vi "Test Cannot Open View Before Start.vi"(8 "error in (no error)":errorcluster, 11 "View Test In":refnum<class "View Dev Test.lvclass">) -> (0 "error out":errorcluster, 3 "View Test Out":refnum<class "View Dev Test.lvclass">)   [LabVIEW 2020, in "View Dev Test.lvclass"]
uses:
  View Dev Test.lvclass
  C:/Program Files (x86)/National Instruments/LabVIEW 2020/vi.lib/Astemes/LUnit/Test Case.lvclass
  source/Framework/Process/Process.lvclass/Process.ctl
  source/Framework/View/View.lvclass/View.ctl
  <vilib>/Astemes/LUnit/Test Case.lvclass/Test Case.ctl
  <vilib>/Astemes/LUnit/LUnit Assertion Result.lvclass/LUnit Assertion Result.ctl
  <vilib>/Astemes/LUnit/LUnit Test Case Result.lvclass/LUnit Test Case Result.ctl
  <vilib>/Astemes/LUnit/LUnit Method Result.lvclass/LUnit Method Result.ctl
  source/Framework/Process/Protected/Messaging/Enqueue Message.vi
  source/Framework/View/Public/Get View VI Reference.vi
  source/Framework/Process/Public/Lifecycle/Get Lifecycle State.vi
  <vilib>/Astemes/LUnit/Palette/Fail.vi
  <vilib>/Astemes/LUnit/Palette/Pass.vi
  <vilib>/Astemes/LUnit/Set Assertion Type.vi
  source/Framework/Process/Private/SubVIs/Handle Debug Data.vi
  source/Framework/Process/Protected/Messaging/Request Message.vi
  <vilib>/Utility/error.llb/Clear Errors.vi
  <vilib>/Astemes/LUnit/Add test result.vi
  <vilib>/Astemes/LUnit/LUnit Write Passed.vi
  <vilib>/Astemes/LUnit/LUnit Write Message.vi
  <vilib>/Astemes/LUnit/LUnit Write Description.vi
  <vilib>/Astemes/LUnit/LUnit Write Assertion Type.vi
  source/Framework/Logging/Log Debug.vi
  <vilib>/AdvancedString/1D String Array to Delimited String.vi
  <vilib>/Utility/High Resolution Relative Seconds.vi
  source/Framework/Process/Private/SubVIs/Enqueue Request Message.vi
  <vilib>/Astemes/LUnit/LUnit Record Assertion Result.vi
  <vilib>/Astemes/LUnit/LUnit Aggregate Assertion Results.vi
  <vilib>/Astemes/LUnit/Assertion Result/LUnit Read Status.vi
  <vilib>/Astemes/LUnit/LUnit Read Message.vi
  <vilib>/Astemes/LUnit/LUnit Read Description.vi
  <vilib>/Astemes/LUnit/Method Result/LUnit Merge Status.vi
  <vilib>/Astemes/LUnit/LUnit Concatenate result strings.vi
  source/Framework/View/View.lvclass
  C:/Git/astemes-triarc-framework/source/Framework/Process/Process.lvclass
  <vilib>/Utility/error.llb/Error Cluster From Error Code.vi
  source/Framework/Process/Public/Read Name.vi
  source/Framework/Process/Private/SubVIs/Wait for Response Message.vi
  <vilib>/Astemes/LUnit/LUnit Assertion Result.lvclass
  <vilib>/Astemes/LUnit/Test Case.lvclass
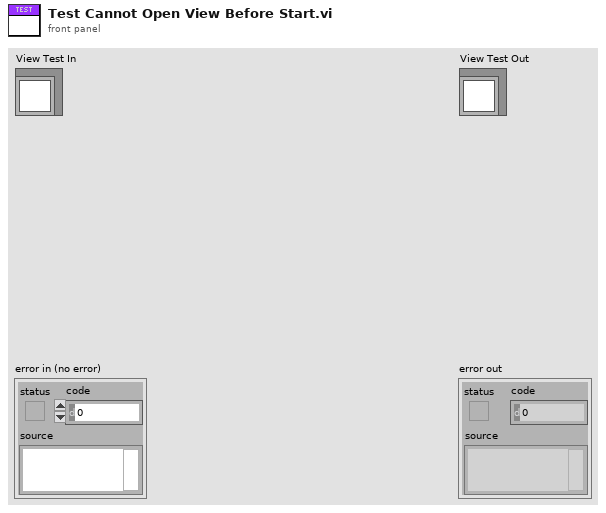
[diagram p1: front panel]
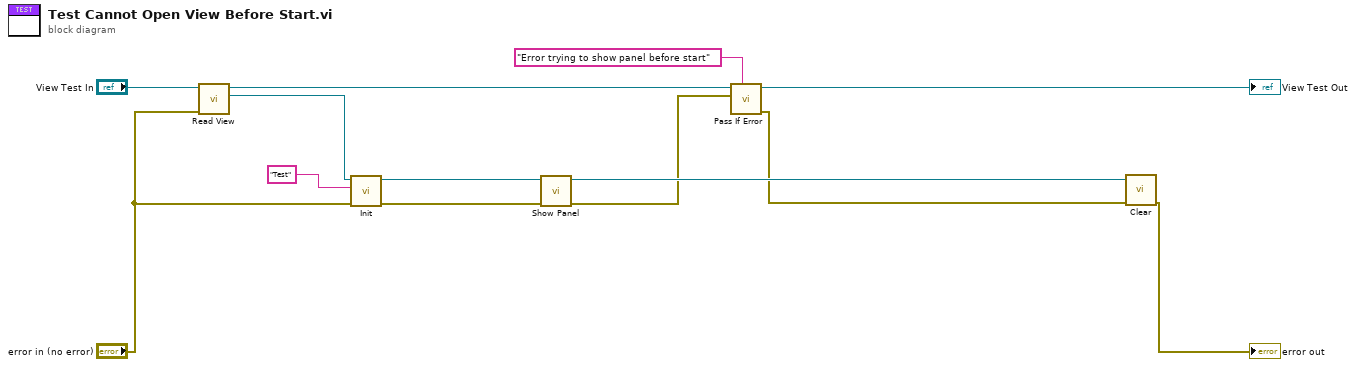
[diagram p0: block diagram]
diagram:
  n1 = call "Read View.vi"("error in (no error)"="error in (no error)", "View Test In"="View Test In") -> ("View"=w12:refnum<class "View.lvclass">, "View Test Out"=w13:refnum<class "View Dev Test.lvclass">)  [unwired: 7 in, 1 out]
  n2 = call-dynamic "Init.vi"("error in (no error)"="error in (no error)", "Name"="Test", "View In"=w12) -> ("error out"=w6:errorcluster, "View Out"=w7:refnum<class "View.lvclass">)  [unwired: 7 in]
  n3 = call "Show Panel.vi"("error in (no error)"=w6, "View In"=w7) -> ("error out"=w3:errorcluster, "View Out"=w5:refnum<class "View.lvclass">)  [unwired: 8 in]
  n4 = call <vilib>:"Pass If Error.vi"("Description"="Error trying to show panel before start", "Assert error"=w3, "LUnit Test Case In"=w13) -> ("error out"=w1:errorcluster, "LUnit Test Case Out"=→"View Test Out":refnum<class "View Dev Test.lvclass">)  [unwired: 7 in]
  n5 = call-dynamic "Clear.vi"("error in (no error)"=w1, "View In"=w5) -> ("error out"=→"error out":errorcluster)  [unwired: 9 in]
